vi "SndPB - Stop.vi"(0 "reference in":refnum<class "GSwFormDSP.lvclass">, 5 "error in (no error)":errorcluster) -> (13 "Cursor Init Location (s)":dbl, 14 "reference out":refnum<class "GSwFormDSP.lvclass">, 19 "error out":errorcluster)   [LabVIEW 2020, in "GSwFormDSP.lvclass"]
uses:
  GSwFormDSP.lvclass
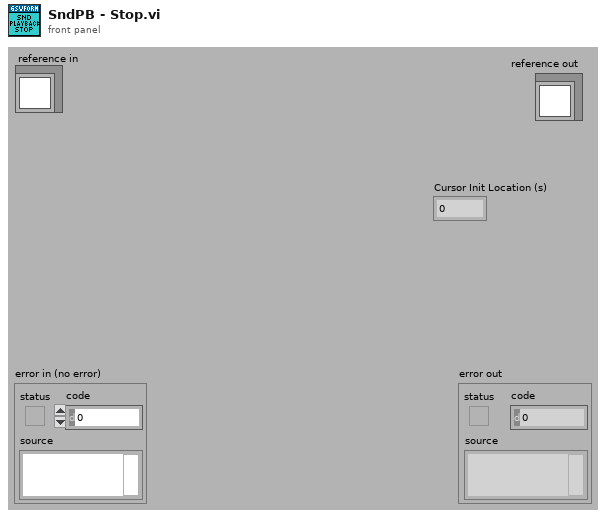
[diagram p1: front panel]
types:
  T1 = typedef "GSwFormDSP.lvclass/Sound Playback.ctl" = cluster{"Timer start (ms)":u32, "task ID":T2, "Cursor Init Location (s)":dbl, "SC Volume":dbl}
  T2 = typedef "Sound Output Task ID.ctl" = u32
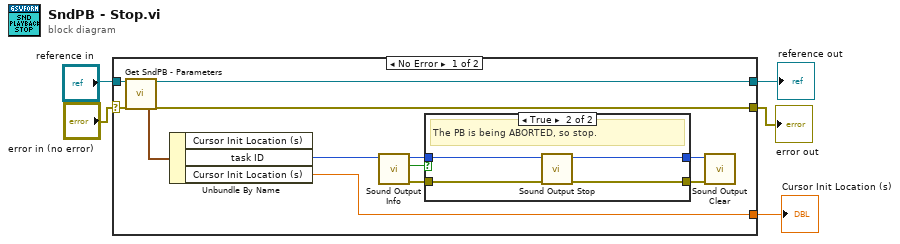
[diagram p0: block diagram]
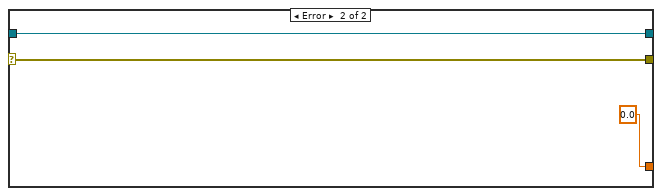
[diagram p3: hidden frame]
diagram:
  n1 = case shown="No Error" "error in (no error)" {
    selector: "error in (no error)" -> [w10 w26]
    tunnel: [w7 w26] -> w4
    tunnel: [w11 w25] -> w2
    tunnel: "reference in" -> [w12 w25]
    tunnel: [w6 0.0 ("Cursor Init Location (s)")] -> w1
    frame No Error {
      n2 = call "Get SndPB - Parameters.vi"("reference in"=w12, "error in (no error)"=w10) -> ("Sound Playback"=w9:T1, "reference out"=w11:refnum<class "GSwFormDSP.lvclass">, "error out"=w7:errorcluster)  [unwired: 15 in]
      n3 = Unbundle By Name(w9) -> ("task ID"=w8:T2, "Cursor Init Location (s)"=w6:dbl)  [unwired: 1 out]
      n4 = call <vilib>:"Sound Output Info.vi"("task ID"=w8) -> ("error out"=w16:errorcluster, "is playing?"=w17:bool, "task ID out"=w14:T2)  [unwired: 7 in, 1 out]
      n5 = case shown="True" w17 {
        tunnel: w16 -> [w18 w22]
        tunnel: [w18 w21] -> w15
        tunnel: w14 -> [w19 w23]
        tunnel: [w19 w20] -> w13
        frame False {
          # "Sound PB terminated normally"
        }
        frame True {
          # "The PB is being ABORTED, so stop."
          n6 = call <vilib>:"Sound Output Stop.vi"("error in (no error)"=w22, "task ID"=w23) -> ("error out"=w21:errorcluster, "task ID out"=w20:T2)  [unwired: 8 in]
        }
      }
      n7 = call <vilib>:"Sound Output Clear.vi"("error in (no error)"=w15, "task ID"=w13) -> ()  [unwired: 9 in, 1 out]
    }
    frame Error {
    }
  }
  "error out" <- w4
  "reference out" <- w2
  "Cursor Init Location (s)" <- w1
